vi "Run Deployment.vi"(8 "error in (no error)":errorcluster, 10 "Targets in":T3 {"Filtered Targets"."IP Mode" items=["Static"=1, "DHCP/Link-Local"=2, "Link-Local Only"=4, "DHCP Only"=8]}, 11 "Ctl Refs in":T6) -> (0 "error out":errorcluster, 1 "Execution State out":T1, 2 "Targets out":T3 {"Filtered Targets"."IP Mode" items=["Static"=1, "DHCP/Link-Local"=2, "Link-Local Only"=4, "DHCP Only"=8]}, 3 "Ctl Refs out":T6, 4 "Buttons out":T2)   [LabVIEW 2013]
uses:
  Controls/Refs.ctl
  Controls/Button Refs.ctl
  Controls/Tab Ctl Refs.ctl
  types/TabStateType.ctl
  Controls/Indicator Refs.ctl
  Controls/Slider Refs.ctl
  Controls/Control Refs.ctl
  Controls/Targets.ctl
  Controls/Detected.ctl
  types/MAX Sys Cfg Target Information.ctl
  types/ButtonStateType.ctl
  types/ExecutionStateType.ctl
panel:
  in  "Stop":bool
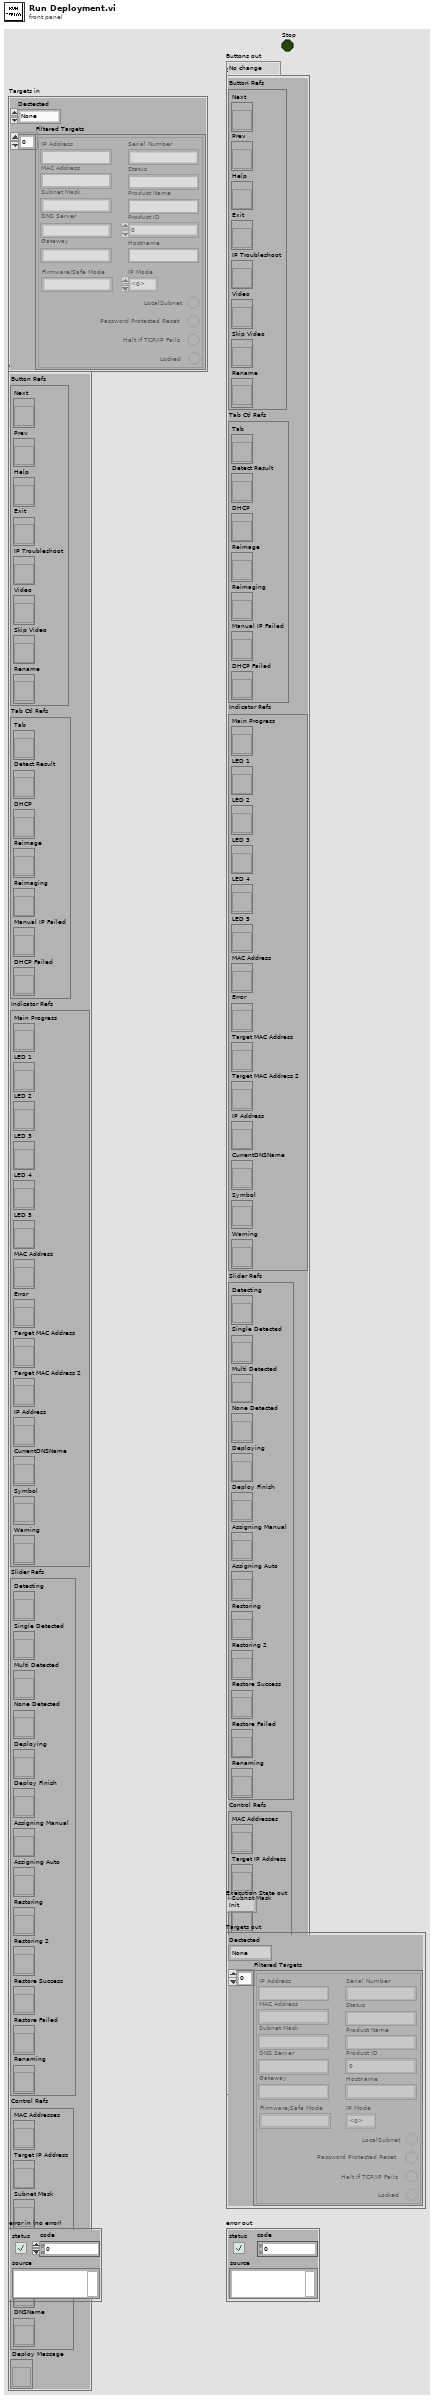
[diagram p1: front panel]
types:
  T1 = typedef "ExecutionStateType.ctl" = enum16{"Init", "Welcome", "Idle", "Detect", "Run Detection", "Detect Fail", "Detect One", "Detect Mult", "Deploy", "DHCP", "Static IP", "Run Deployment", "Connect Verify", "Exit", "Video Wait", "Success", "Troubleshoot", "Troubleshoot 2", "RenameDNS"}
  T2 = typedef "ButtonStateType.ctl" = enum16{"No change", "No Next", "No Prev", "All Disabled", "All Enabled", "Exit Only"}
  T3 = typedef "Targets.ctl" = cluster{"Dectected":T4, "Filtered Targets":T5[]}
  T4 = typedef "Detected.ctl" = enum16{"None", "Failed", "Single", "Multi"}
  T5 = typedef "MAX Sys Cfg Target Information.ctl" = cluster{"MAC Address":string, "IP Address":string, "Status":string, "Product Name":string, "Hostname":string, "Firmware/Safe Mode":string, "Subnet Mask":string, "Gateway":string, "DNS Server":string, "Serial Number":string, "Product ID":u32, "Locked ":bool, "LocalSubnet":bool, "Halt If TCP/IP Fails":bool, "Password Protected Reset":bool, "IP Mode":i32}
  T6 = typedef "Refs.ctl" = cluster{"Button Refs":T7, "Tab Ctl Refs":T8, "Indicator Refs":T9, "Slider Refs":T10, "Control Refs":T11, "Deploy Message":refnum<vi>}
  T7 = typedef "Button Refs.ctl" = cluster{"Next":refnum<vi>, "Prev":refnum<vi>, "Help":refnum<vi>, "Exit":refnum<vi>, "IP Troubleshoot":refnum<vi>, "Video":refnum<vi>, "Skip Video":refnum<vi>, "Rename":refnum<vi>}
  T8 = typedef "Tab Ctl Refs.ctl" = cluster{"Tab":refnum<vi>, "Detect Result":refnum<vi>, "DHCP":refnum<vi>, "Reimage":refnum<vi>, "Reimaging":refnum<vi>, "Manual IP Failed":refnum<vi>, "DHCP Failed":refnum<vi>}
  T9 = typedef "Indicator Refs.ctl" = cluster{"Main Progress":refnum<vi>, "LED 1":refnum<vi>, "LED 2":refnum<vi>, "LED 3":refnum<vi>, "LED 4":refnum<vi>, "LED 5":refnum<vi>, "MAC Address":refnum<vi>, "Error":refnum<vi>, "Target MAC Address":refnum<vi>, "Target MAC Address 2":refnum<vi>, "IP Address":refnum<vi>, "CurrentDNSName":refnum<vi>, "Symbol":refnum<vi>, "Warning":refnum<vi>}
  T10 = typedef "Slider Refs.ctl" = cluster{"Detecting":refnum<vi>, "Single Detected":refnum<vi>, "Multi Detected":refnum<vi>, "None Detected":refnum<vi>, "Deploying":refnum<vi>, "Deploy Finish":refnum<vi>, "Assigning Manual":refnum<vi>, "Assigning Auto":refnum<vi>, "Restoring":refnum<vi>, "Restoring 2":refnum<vi>, "Restore Success":refnum<vi>, "Restore Failed":refnum<vi>, "Renaming":refnum<vi>}
  T11 = typedef "Control Refs.ctl" = cluster{"MAC Addresses":refnum<vi>, "Target IP Address":refnum<vi>, "Subnet Mask":refnum<vi>, "DNS IP":refnum<vi>, "Default Gateway":refnum<vi>, "DNSName":refnum<vi>}
  T12 = typedef "TabStateType.ctl" = enum32{"Welcome", "Instructions", "Detect", "Run Detection", "Detect Result", "Deploy", "Run Deployment", "Connect Verify", "Success", "DHCP", "Troubleshoot", "System Restore", "Error", "Video", "Rename"}
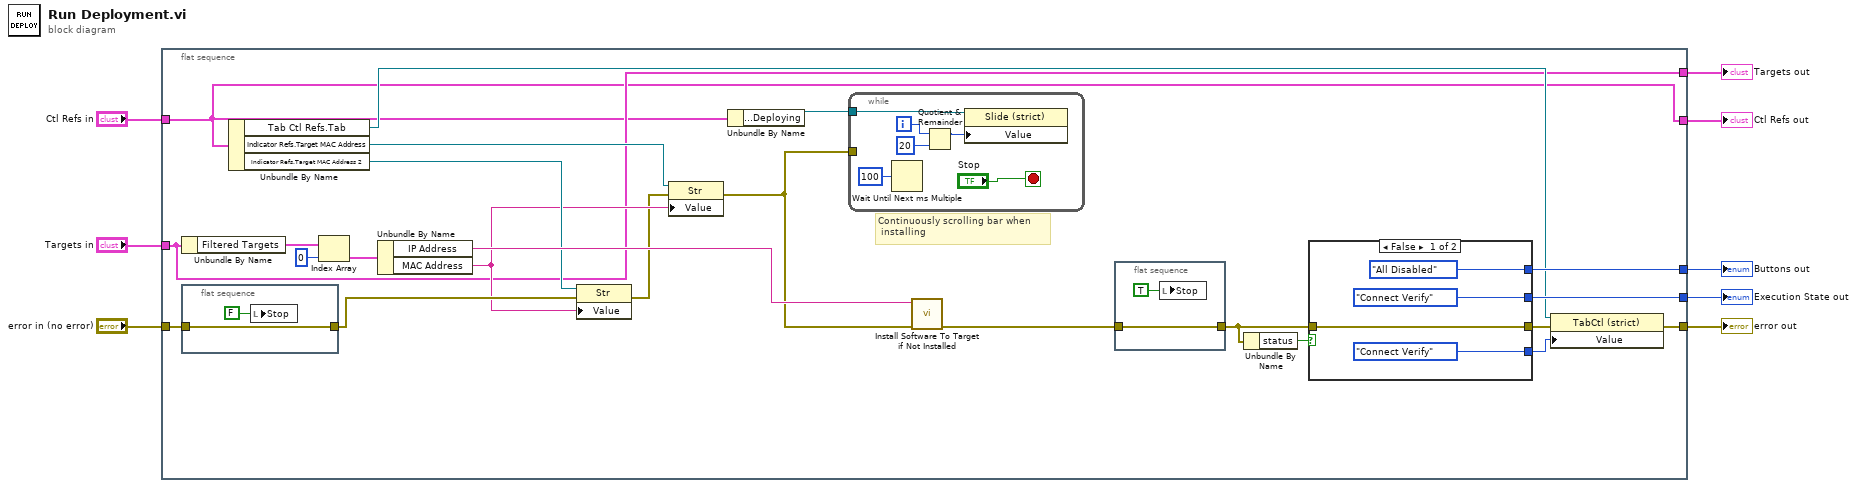
[diagram p0: block diagram]
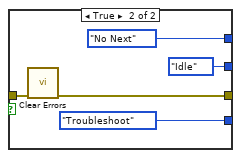
[diagram p2: hidden frame]
diagram:
  n1 = flat-sequence {
    tunnel: [w31] -> w1
    tunnel: "error in (no error)" -> [w28]
    tunnel: [w24] -> w3
    tunnel: [w23] -> w4
    tunnel: "Targets in" -> [w14]
    tunnel: "Ctl Refs in" -> [w12]
    tunnel: [w14] -> w7
    tunnel: [w12] -> w8
    frame #0 {
      # "Continuously scrolling bar when\n installing"
      n2 = Unbundle By Name(w14) -> ("Filtered Targets"=w19:T5[])
      n3 = flat-sequence {
        tunnel: w28 -> [w48]
        tunnel: [w48] -> w18
        frame #0 {
          n4 = local write "Stop"(FALSE) -> ()
        }
      }
      n5 = Unbundle By Name(w12) -> ("Tab Ctl Refs.Tab"=w20:refnum<vi>, "Indicator Refs.Target MAC Address"=w16:refnum<vi>, "Indicator Refs.Target MAC Address 2"=w17:refnum<vi>)
      n6 = Index Array(array=w19, index=0) -> (element=w29:T5)
      n7 = Unbundle By Name(w29) -> ("IP Address"=w21:string, "MAC Address"=w15:string)
      n8 = property class="Str"(reference=w17, error in=w18, "Value"=w15) -> (error out=w10:errorcluster)  [unwired: 1 out]
      n9 = property class="Str"(reference=w16, error in=w10, "Value"=w15) -> (error out=w9:errorcluster)  [unwired: 1 out]
      n10 = Unbundle By Name(w12) -> ("Slider Refs.Deploying"=w11:refnum<vi>)
      n11 = while {
        tunnel: w11 -> [w34]
        tunnel: w9 -> [_]
        i -> [w35]
        stop <- "Stop" stop-if-true
        n12 = Wait Until Next ms Multiple(millisecond multiple=u32 100 ("milliseconds to wait")) -> ()  [unwired: 1 out]
        n13 = Quotient & Remainder(x=w35, y=20) -> (x-y*floor(x/y)=w33:i32)  [unwired: 1 out]
        n14 = property class="Slide (strict)"(reference=w34, "Value"=w33) -> ()  [unwired: 1 in, 2 out]
      }
      n15 = call "Install Software To Target if Not Installed.vi"("error in (no error)"=w9, "MAC Address"=w21) -> ("error out"=w13:errorcluster)  [unwired: 8 in, 1 out]
      n16 = flat-sequence {
        tunnel: w13 -> [w50]
        tunnel: [w50] -> w27
        frame #0 {
          n17 = local write "Stop"(TRUE) -> ()
        }
      }
      n18 = Unbundle By Name(w27) -> ("status"=w22:bool)
      n19 = case shown="False" w22 {
        tunnel: w27 -> [w41 w46]
        tunnel: [w41 w45] -> w25
        tunnel: [TabStateType."Connect Verify" ("Tab Control") TabStateType."Troubleshoot" ("Tab Control")] -> w26
        tunnel: [ExecutionStateType."Connect Verify" ("Enum") ExecutionStateType."Idle" ("Enum")] -> w24
        tunnel: [ButtonStateType."All Disabled" ("Enum") ButtonStateType."No Next" ("Enum")] -> w23
        frame False {
        }
        frame True {
          n20 = call <vilib>:"Clear Errors.vi"("error in (no error)"=w46) -> ("error out"=w45:errorcluster)  [unwired: 6 out]
        }
      }
      n21 = property on="Property Node" class="TabCtl (strict)"(reference=w20, error in=w25, "Value"=w26) -> (error out=w31:errorcluster)  [unwired: 1 out]
    }
  }
  "Ctl Refs out" <- w8
  "Targets out" <- w7
  "Buttons out" <- w4
  "Execution State out" <- w3
  "error out" <- w1
